vi "Check Food Collision.vi"(11 "Map In":u32[][](array[numeric])) -> (1 "X Position":i32, 2 "Y Position":i32, 3 "Map Out":u32[][](array[numeric]), 4 "Collision?":bool)   [LabVIEW 2014]
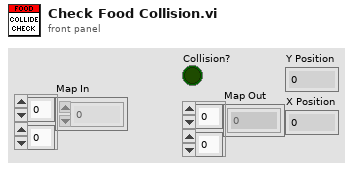
[diagram p1: front panel]
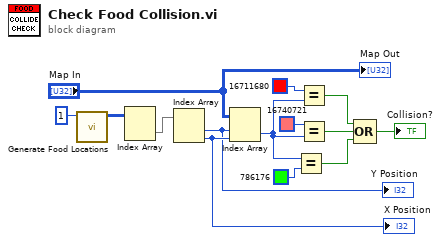
[diagram p0: block diagram]
diagram:
  n1 = call "Generate Food Locations.vi"("Num Food"=1) -> ("Food Array"=w6:i32[][])  [unwired: 10 in]
  n2 = Index Array(array=w6) -> (element=w7:i32[])  [unwired: 2 in]
  n3 = Index Array(array=w7) -> (element #1=w9:i32, element #2=w10:i32)  [unwired: 2 in]
  "Y Position" <- w9
  "X Position" <- w10
  n4 = Index Array(array="Map In", index (row)=w9, index (col)=w10) -> (element=w14:u32)
  n5 = Equal?(x=w14, y=u32 786176) -> (x = y?=w2:bool)
  n6 = Equal?(x=u32 16711680, y=w14) -> (x = y?=w4:bool)
  n7 = Equal?(x=u32 16740721, y=w14) -> (x = y?=w3:bool)
  n8 = Compound Arithmetic op=OR(w4, w3, w2) -> (→"Collision?":bool)
  "Map Out" <- "Map In"
